vi "2048_cal_all.vi"(9 "score in":i32, 10 "VKey in":T1, 11 "matrix":i32[][](array[numeric])) -> (0 "valid move":bool, 1 "score out":i32, 2 "VKey out":T1, 3 "matrix out":i32[][](array[numeric]))   [LabVIEW 2022 SP3]
uses:
  <vilib>/event_ctls.llb/eventvkey.ctl
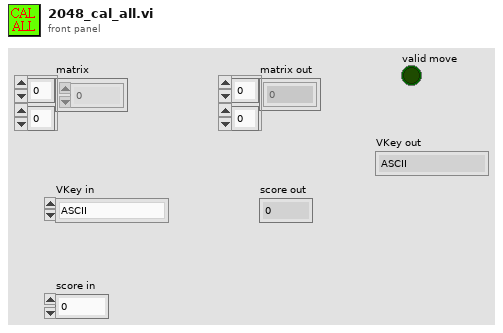
[diagram p1: front panel]
types:
  T1 = typedef "eventvkey.ctl" = enum16{"ASCII", "Enter", "Return", "Shift", "Ctrl", "Alt", "Cmd", "Opt", "Caps", "NumLock", "Clear", "Break", "Up", "Down", "Left", "Right", "Insert", "Delete", "Home", "End", "PageUp", "PageDown", "Escape", "Help", "Pause", "ScrollLock", "F1", "F2", "F3", "F4", "F5", "F6", "F7", "F8", "F9", "F10", "F11", "F12", "F13", "F14", "F15", "F16", "F17", "F18", "F19", "F20", "F21", "F22", "F23", "F24", "Play", "VolumeUp", "VolumeDown", "Mute", "Two Byte Char"}
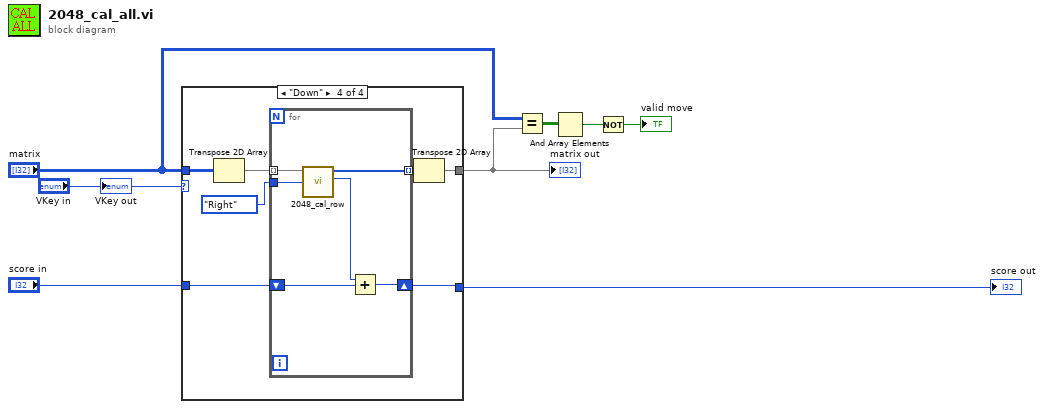
[diagram p0: block diagram]
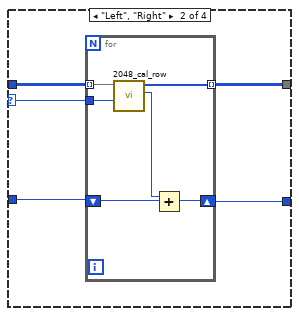
[diagram p3: hidden frame]
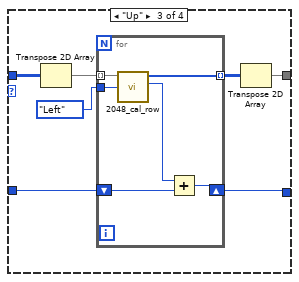
[diagram p4: hidden frame]
diagram:
  n1 = case shown="\"Down\"" "VKey in" {
    selector: "VKey in" -> [_ w13 _ _]
    tunnel: "matrix" -> [w10 w15 w28 w41]
    tunnel: [w10 w14 w25 w38] -> w5
    tunnel: "score in" -> [w9 w12 w23 w36]
    tunnel: [w9 w11 w22 w35] -> w7
    frame "ASCII", Default {
    }
    frame "Left", "Right" {
      n2 = for {
        tunnel: w13 -> [w21]
        tunnel: w15 -> [w20] mode=indexing
        tunnel: [w19] -> w14 mode=indexing
        shift-right: [w16] -> w11
        shift-left: w12 -> [w17]
        n3 = call "2048_cal_row.vi"("VKey"=w21, "Array in"=w20) -> ("score_add"=w18:i32, "Array out"=w19:i32[])  [unwired: 8 in]
        n4 = Add(x=w18, y=w17) -> (x+y=w16:i32)
      }
    }
    frame "Up" {
      n5 = Transpose 2D Array(2D array=w28) -> (transposed array=w27:i32[][])
      n6 = for {
        tunnel: w27 -> [w34] mode=indexing
        tunnel: [w33] -> w26 mode=indexing
        tunnel: eventvkey."Left" ("VKey") -> [w32]
        shift-right: [w31] -> w22
        shift-left: w23 -> [w30]
        n7 = call "2048_cal_row.vi"("VKey"=w32, "Array in"=w34) -> ("score_add"=w29:i32, "Array out"=w33:i32[])  [unwired: 8 in]
        n8 = Add(x=w29, y=w30) -> (x+y=w31:i32)
      }
      n9 = Transpose 2D Array(2D array=w26) -> (transposed array=w25:i32[][])
    }
    frame "Down" {
      n10 = Transpose 2D Array(2D array=w41) -> (transposed array=w40:i32[][])
      n11 = for {
        tunnel: w40 -> [w47] mode=indexing
        tunnel: [w46] -> w39 mode=indexing
        tunnel: eventvkey."Right" ("VKey") -> [w45]
        shift-right: [w44] -> w35
        shift-left: w36 -> [w43]
        n12 = call "2048_cal_row.vi"("VKey"=w45, "Array in"=w47) -> ("score_add"=w42:i32, "Array out"=w46:i32[])  [unwired: 8 in]
        n13 = Add(x=w42, y=w43) -> (x+y=w44:i32)
      }
      n14 = Transpose 2D Array(2D array=w39) -> (transposed array=w38:i32[][])
    }
  }
  "matrix out" <- w5
  "score out" <- w7
  n15 = Equal?(x="matrix", y=w5) -> (x = y?=w3:bool[][])
  n16 = And Array Elements(Boolean array=w3) -> (logical AND=w2:bool)
  n17 = Not(x=w2) -> (.not. x?=→"valid move":bool)
  "VKey out" <- "VKey in"
